vi "CODMn流程步骤.vi"() -> ()   [LabVIEW 2016]
panel:
  out "步骤时间/秒":T1={"步骤1时间"=2, "步骤2时间"=4, "步骤3时间"=2, "步骤4时间"=5, "步骤5时间"=6, "步骤6时间"=3, "步骤7时间"=4, "步骤8时间"=7, "步骤9时间"=8, "步骤10时间"=6}
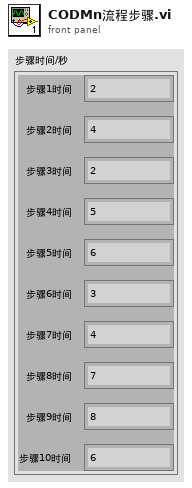
[diagram p1: front panel]
types:
  T1 = cluster{"步骤1时间":i32, "步骤2时间":i32, "步骤3时间":i32, "步骤4时间":i32, "步骤5时间":i32, "步骤6时间":i32, "步骤7时间":i32, "步骤8时间":i32, "步骤9时间":i32, "步骤10时间":i32}
  T2 = enum16{"步骤1", "步骤2", "步骤3", "步骤4", "步骤5", "步骤6", "步骤7", "步骤8", "步骤9", "步骤10"}
  T3 = cluster{"因子编码":u32, "单位":u16, "标样参考值":sgl, "水样数据时间":timestamp, "水样实测值":sgl, "水样数据标识":string, "标样数据时间":timestamp, "标样实测值":sgl, "标样数据标识":string, "空白数据时间":timestamp, "空白实测值":sgl, "空白数据标识":string, "零点核查数据时间":timestamp, "零点核查实测值":sgl, "零点核查数据标识":string, "跨度核查数据时间":timestamp, "跨度核查实测值":sgl, "跨度核查数据标识":string, "加标回收数据时间":timestamp, "加标回收实测值":sgl, "加标回收数据标识":string, "平行样数据时间":timestamp, "平行样实测值":sgl, "平行样数据标识":string}
  T4 = cluster{"系统时间":timestamp, "工作状态":u16, "测量模式":u16, "告警代码":enum16{"无告警", "缺试剂告警", "缺水样告警", "缺蒸馏水告警", "缺标液告警", "仪表漏液告警", "标定异常告警", "超量程告警", "加热异常", "低试剂预警", "超上限告警", "超下限告警", "仪表内部其他异常", "滴定异常告警", "电极异常告警", "量程切换告警", "参数设置告警", "PH电极电位异常", "电导率电极异常", "浊度光度异常", "溶解氧电极异常", "溶解氧光强异常", "温度异常告警", "PH异常告警", "溶解氧异常告警", "电导率异常告警", "浊度异常告警", "叶绿素异常告警", "藻密度异常告警", "蓝绿藻异常告警", "ORP异常告警", "氨氮异常告警", "清洁刷异常告警", "SD卡异常告警", "蓝牙异常告警", "Wifi异常告警", "流程异常告警"}, "故障代码":enum16{"无故障", "电机故障", "温度故障", "通讯故障", "滴定故障"}, "日志代码":u16, "软件版本":u16, "F0":sgl, "F1":sgl, "F2":sgl, "F3":sgl, "T":sgl, "H":sgl, "id":u16, "flowid":u16, "量程":u16}
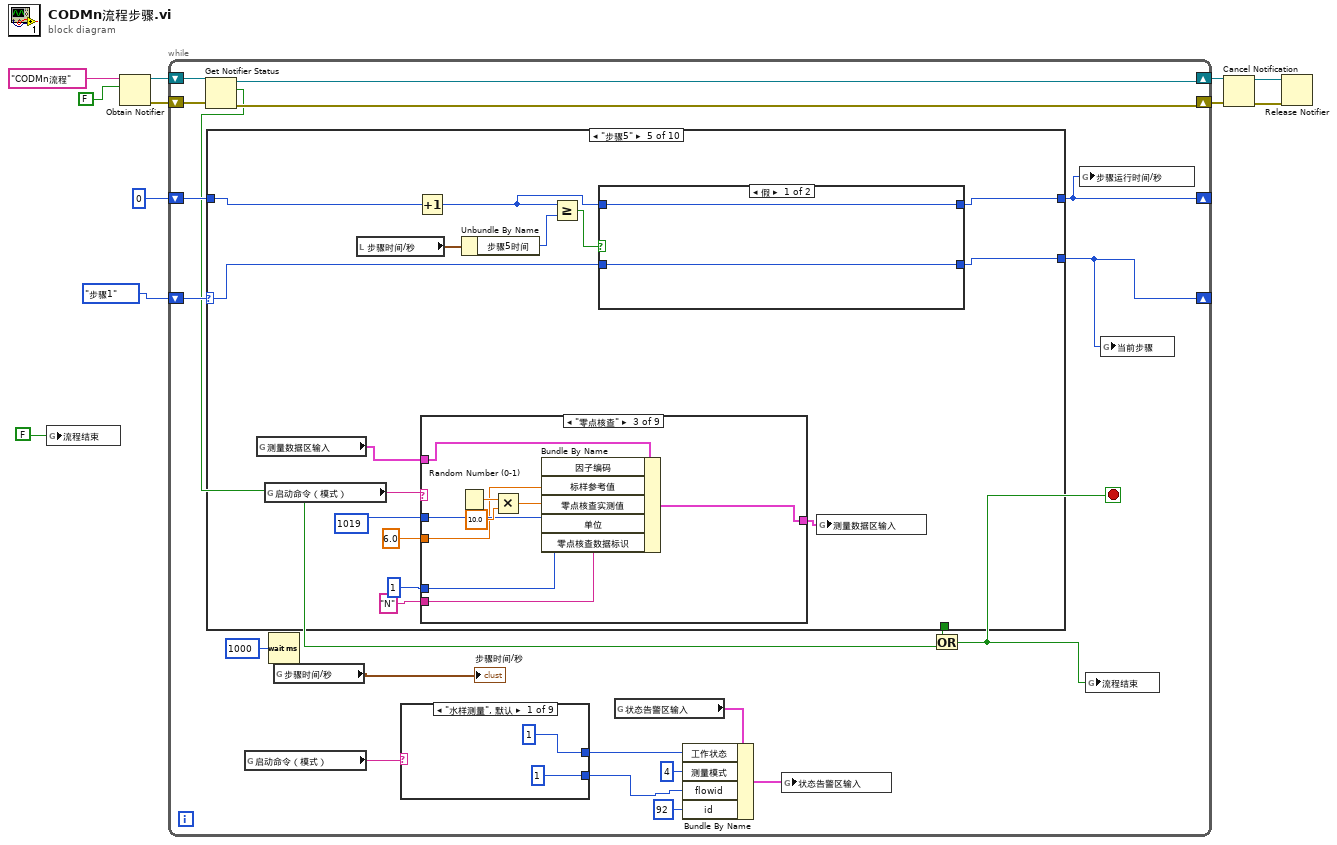
[diagram p0: block diagram]
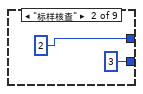
[diagram p2: hidden frame]
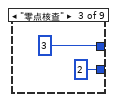
[diagram p3: hidden frame]
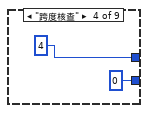
[diagram p4: hidden frame]
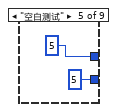
[diagram p5: hidden frame]
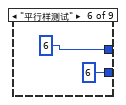
[diagram p6: hidden frame]
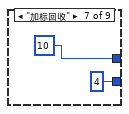
[diagram p7: hidden frame]
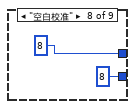
[diagram p8: hidden frame]
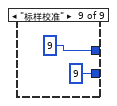
[diagram p9: hidden frame]
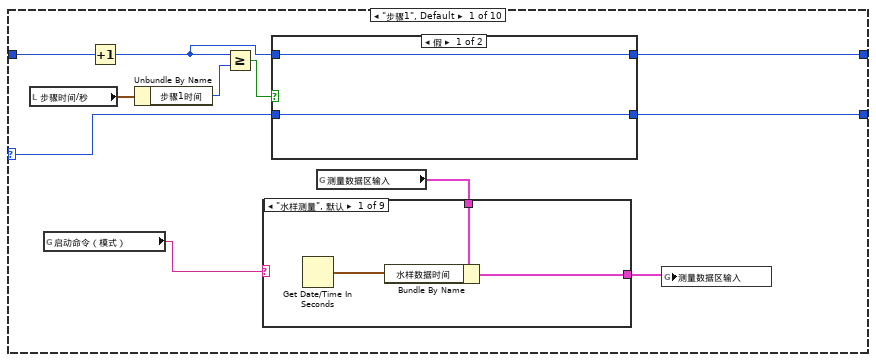
[diagram p10: hidden frame]
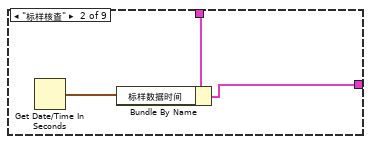
[diagram p11: hidden frame]
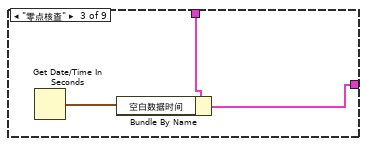
[diagram p12: hidden frame]
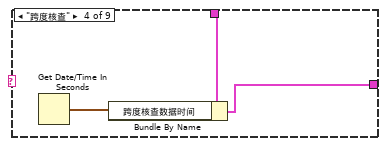
[diagram p13: hidden frame]
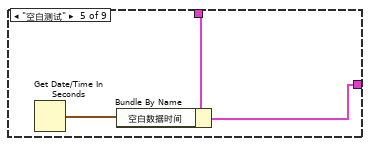
[diagram p14: hidden frame]
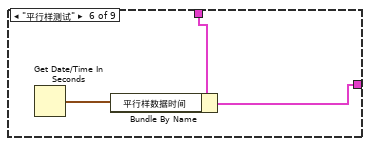
[diagram p15: hidden frame]
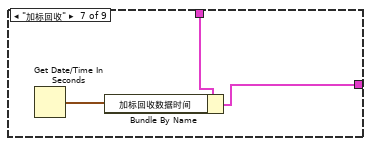
[diagram p16: hidden frame]
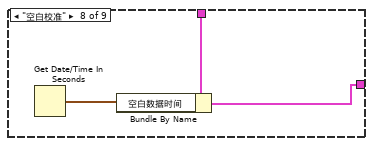
[diagram p17: hidden frame]
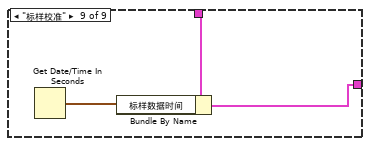
[diagram p18: hidden frame]
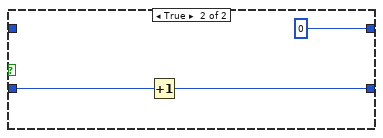
[diagram p19: hidden frame]
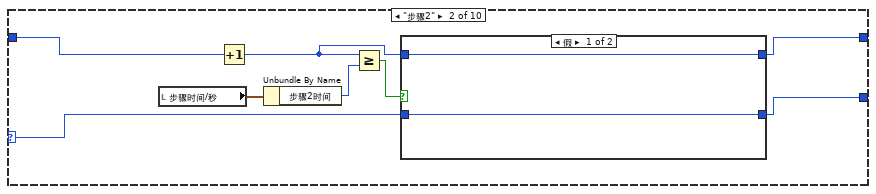
[diagram p20: hidden frame]
diagram:
  n1 = global write "CODMn全局.vi" "流程结束"(FALSE ("流程结束")) -> ()
  n2 = Obtain Notifier(name (unnamed)="CODMn流程" ("名称（未命名）"), notification data type=FALSE) -> (notifier out=w7:refnum<notifier>, error out=w6:errorcluster)  [unwired: 2 in, 1 out]
  n3 = while {
    shift-right: [w16] -> _
    shift-left: T2."步骤1" -> [w31]
    shift-right: [w17] -> _
    shift-left: 0 -> [w29]
    shift-right: [w25] -> w3
    shift-left: w7 -> [w27]
    shift-right: [w24] -> w2
    shift-left: w6 -> [w26]
    stop <- w18 stop-if-true
    n4 = Get Notifier Status(notifier=w27, error in (no error)=w26) -> (notifier out=w25:refnum<notifier>, current notification=w23:bool, error out=w24:errorcluster)  [unwired: 2 out]
    n5 = case shown="\"步骤5\"" w31 {
      selector: w31 -> [w54 w95 w108 w121 w141 w235 w248 w261 w274 w288]
      tunnel: [_ _ _ _ _ _ _ _ _ w285] -> w28
      tunnel: w29 -> [w60 w96 w109 w122 w142 w236 w249 w262 w275 w289]
      tunnel: [w56 w94 w107 w120 w140 w234 w247 w260 w273 w287] -> w17
      tunnel: [w53 w93 w106 w119 w139 w233 w246 w259 w272 w286] -> w16
      frame "步骤1", Default {
        n6 = local read "步骤时间/秒"() -> (w59:T1)
        n7 = global read "CODMn全局.vi" "启动命令（模式）"() -> (w50:string)
        n8 = Increment(x=w60) -> (x+1=w55:i32)
        n9 = Unbundle By Name(w59) -> ("步骤1时间"=w58:i32)
        n10 = Greater Or Equal?(x=w55, y=w58) -> (x >= y?=w57:bool)
        n11 = case shown="假" w57 {
          tunnel: [w89 0] -> w56
          tunnel: w55 -> [w89 _]
          tunnel: w54 -> [w88 w91]
          tunnel: [w88 w90] -> w53
          frame False {
          }
          frame True {
            n12 = Increment(x=w91) -> (x+1=w90:T2)
          }
        }
        n13 = global read "CODMn全局.vi" "测量数据区输入"() -> (w52:T3)
        n14 = case shown="\"水样测量\", 默认" w50 {
          tunnel: w52 -> [w62 w65 w68 w71 w74 w77 w80 w83 w86]
          tunnel: [w61 w64 w67 w70 w73 w76 w79 w82 w85] -> w51
          frame "水样测量", Default {
            n15 = Get Date/Time In Seconds() -> (seconds since 1Jan1904=w63:timestamp)
            n16 = Bundle By Name(cluster=w62, "水样数据时间"=w63) -> (w61:T3)
          }
          frame "标样核查" {
            n17 = Get Date/Time In Seconds() -> (seconds since 1Jan1904=w66:timestamp)
            n18 = Bundle By Name(cluster=w65, "标样数据时间"=w66) -> (w64:T3)
          }
          frame "零点核查" {
            n19 = Get Date/Time In Seconds() -> (seconds since 1Jan1904=w69:timestamp)
            n20 = Bundle By Name(cluster=w68, "空白数据时间"=w69) -> (w67:T3)
          }
          frame "跨度核查" {
            n21 = Get Date/Time In Seconds() -> (seconds since 1Jan1904=w72:timestamp)
            n22 = Bundle By Name(cluster=w71, "跨度核查数据时间"=w72) -> (w70:T3)
          }
          frame "空白测试" {
            n23 = Get Date/Time In Seconds() -> (seconds since 1Jan1904=w75:timestamp)
            n24 = Bundle By Name(cluster=w74, "空白数据时间"=w75) -> (w73:T3)
          }
          frame "平行样测试" {
            n25 = Get Date/Time In Seconds() -> (seconds since 1Jan1904=w78:timestamp)
            n26 = Bundle By Name(cluster=w77, "平行样数据时间"=w78) -> (w76:T3)
          }
          frame "加标回收" {
            n27 = Get Date/Time In Seconds() -> (seconds since 1Jan1904=w81:timestamp)
            n28 = Bundle By Name(cluster=w80, "加标回收数据时间"=w81) -> (w79:T3)
          }
          frame "空白校准" {
            n29 = Get Date/Time In Seconds() -> (seconds since 1Jan1904=w84:timestamp)
            n30 = Bundle By Name(cluster=w83, "空白数据时间"=w84) -> (w82:T3)
          }
          frame "标样校准" {
            n31 = Get Date/Time In Seconds() -> (seconds since 1Jan1904=w87:timestamp)
            n32 = Bundle By Name(cluster=w86, "标样数据时间"=w87) -> (w85:T3)
          }
        }
        n33 = global write "CODMn全局.vi" "测量数据区输入"(w51) -> ()
      }
      frame "步骤2" {
        n34 = local read "步骤时间/秒"() -> (w100:T1)
        n35 = Increment(x=w96) -> (x+1=w97:i32)
        n36 = Unbundle By Name(w100) -> ("步骤2时间"=w99:i32)
        n37 = Greater Or Equal?(x=w97, y=w99) -> (x >= y?=w98:bool)
        n38 = case shown="假" w98 {
          tunnel: [w102 0] -> w94
          tunnel: w97 -> [w102 _]
          tunnel: w95 -> [w101 w104]
          tunnel: [w101 w103] -> w93
          frame False {
          }
          frame True {
            n39 = Increment(x=w104) -> (x+1=w103:T2)
          }
        }
      }
      frame "步骤3" {
        n40 = local read "步骤时间/秒"() -> (w113:T1)
        n41 = Increment(x=w109) -> (x+1=w110:i32)
        n42 = Unbundle By Name(w113) -> ("步骤3时间"=w112:i32)
        n43 = Greater Or Equal?(x=w110, y=w112) -> (x >= y?=w111:bool)
        n44 = case shown="假" w111 {
          tunnel: [w115 0] -> w107
          tunnel: w110 -> [w115 _]
          tunnel: w108 -> [w114 w117]
          tunnel: [w114 w116] -> w106
          frame False {
          }
          frame True {
            n45 = Increment(x=w117) -> (x+1=w116:T2)
          }
        }
      }
      frame "步骤4" {
        n46 = local read "步骤时间/秒"() -> (w126:T1)
        n47 = Increment(x=w122) -> (x+1=w123:i32)
        n48 = Unbundle By Name(w126) -> ("步骤4时间"=w125:i32)
        n49 = Greater Or Equal?(x=w123, y=w125) -> (x >= y?=w124:bool)
        n50 = case shown="假" w124 {
          tunnel: [w128 0] -> w120
          tunnel: w123 -> [w128 _]
          tunnel: w121 -> [w127 w130]
          tunnel: [w127 w129] -> w119
          frame False {
          }
          frame True {
            n51 = Increment(x=w130) -> (x+1=w129:T2)
          }
        }
      }
      frame "步骤5" {
        n52 = global read "CODMn全局.vi" "测量数据区输入"() -> (w133:T3)
        n53 = global read "CODMn全局.vi" "启动命令（模式）"() -> (w134:string)
        n54 = local read "步骤时间/秒"() -> (w146:T1)
        n55 = Increment(x=w142) -> (x+1=w143:i32)
        n56 = case shown="\"零点核查\"" w134 {
          tunnel: u32 1019 ("因子编码") -> [w151 w161 w170 w179 w188 w197 w206 w215 w224]
          tunnel: sgl 6.0 ("标样参考值") -> [w150 w160 w169 w177 w186 w195 w204 w213 w222]
          tunnel: u16 1 ("单位") -> [w149 w159 w168 w178 w187 w196 w205 w214 w223]
          tunnel: "N" -> [w152 w158 w167 w176 w185 w194 w203 w212 w221]
          tunnel: w133 -> [w148 w157 w166 w175 w184 w192 w202 w211 w220]
          tunnel: [w147 w156 w165 w174 w183 w193 w201 w210 w219] -> w132
          frame "水样测量", Default {
            n57 = Random Number (0-1)() -> (number: 0 to 1=w153:dbl)
            n58 = Multiply(x=w153, y=10.0 ("数字(0-1)")) -> (x*y=w155:dbl)
            n59 = Bundle By Name(cluster=w148, "因子编码"=w151, "标样参考值"=w150, "水样实测值"=w155, "单位"=w149, "水样数据标识"=w152) -> (w147:T3)
          }
          frame "标样核查" {
            n60 = Random Number (0-1)() -> (number: 0 to 1=w162:dbl)
            n61 = Multiply(x=w162, y=10.0 ("数字(0-1)")) -> (x*y=w164:dbl)
            n62 = Bundle By Name(cluster=w157, "因子编码"=w161, "标样参考值"=w160, "标样实测值"=w164, "单位"=w159, "标样数据标识"=w158) -> (w156:T3)
          }
          frame "零点核查" {
            n63 = Random Number (0-1)() -> (number: 0 to 1=w171:dbl)
            n64 = Multiply(x=w171, y=10.0 ("数字(0-1)")) -> (x*y=w173:dbl)
            n65 = Bundle By Name(cluster=w166, "因子编码"=w170, "标样参考值"=w169, "零点核查实测值"=w173, "单位"=w168, "零点核查数据标识"=w167) -> (w165:T3)
          }
          frame "跨度核查" {
            n66 = Random Number (0-1)() -> (number: 0 to 1=w180:dbl)
            n67 = Multiply(x=w180, y=10.0 ("数字(0-1)")) -> (x*y=w182:dbl)
            n68 = Bundle By Name(cluster=w175, "因子编码"=w179, "标样参考值"=w177, "跨度核查实测值"=w182, "单位"=w178, "跨度核查数据标识"=w176) -> (w174:T3)
          }
          frame "空白测试" {
            n69 = Random Number (0-1)() -> (number: 0 to 1=w189:dbl)
            n70 = Multiply(x=w189, y=10.0 ("数字(0-1)")) -> (x*y=w191:dbl)
            n71 = Bundle By Name(cluster=w184, "因子编码"=w188, "标样参考值"=w186, "空白实测值"=w191, "单位"=w187, "空白数据标识"=w185) -> (w183:T3)
          }
          frame "平行样测试" {
            n72 = Random Number (0-1)() -> (number: 0 to 1=w198:dbl)
            n73 = Multiply(x=w198, y=10.0 ("数字(0-1)")) -> (x*y=w200:dbl)
            n74 = Bundle By Name(cluster=w192, "因子编码"=w197, "标样参考值"=w195, "平行样实测值"=w200, "单位"=w196, "平行样数据标识"=w194) -> (w193:T3)
          }
          frame "加标回收" {
            n75 = Random Number (0-1)() -> (number: 0 to 1=w207:dbl)
            n76 = Multiply(x=w207, y=10.0 ("数字(0-1)")) -> (x*y=w209:dbl)
            n77 = Bundle By Name(cluster=w202, "因子编码"=w206, "标样参考值"=w204, "加标回收实测值"=w209, "单位"=w205, "加标回收数据标识"=w203) -> (w201:T3)
          }
          frame "空白校准" {
            n78 = Random Number (0-1)() -> (number: 0 to 1=w216:dbl)
            n79 = Multiply(x=w216, y=10.0 ("数字(0-1)")) -> (x*y=w218:dbl)
            n80 = Bundle By Name(cluster=w211, "因子编码"=w215, "标样参考值"=w213, "空白实测值"=w218, "单位"=w214, "跨度核查数据标识"=w212) -> (w210:T3)
          }
          frame "标样校准" {
            n81 = Random Number (0-1)() -> (number: 0 to 1=w225:dbl)
            n82 = Multiply(x=w225, y=10.0 ("数字(0-1)")) -> (x*y=w227:dbl)
            n83 = Bundle By Name(cluster=w220, "因子编码"=w224, "标样参考值"=w222, "标样实测值"=w227, "单位"=w223, "跨度核查数据标识"=w221) -> (w219:T3)
          }
        }
        n84 = Unbundle By Name(w146) -> ("步骤5时间"=w145:i32)
        n85 = Greater Or Equal?(x=w143, y=w145) -> (x >= y?=w144:bool)
        n86 = case shown="假" w144 {
          tunnel: [w229 0] -> w140
          tunnel: w143 -> [w229 _]
          tunnel: w141 -> [w228 w231]
          tunnel: [w228 w230] -> w139
          frame False {
          }
          frame True {
            n87 = Increment(x=w231) -> (x+1=w230:T2)
          }
        }
        n88 = global write "CODMn全局.vi" "测量数据区输入"(w132) -> ()
      }
      frame "步骤6" {
        n89 = local read "步骤时间/秒"() -> (w240:T1)
        n90 = Increment(x=w236) -> (x+1=w237:i32)
        n91 = Unbundle By Name(w240) -> ("步骤6时间"=w239:i32)
        n92 = Greater Or Equal?(x=w237, y=w239) -> (x >= y?=w238:bool)
        n93 = case shown="假" w238 {
          tunnel: [w242 0] -> w234
          tunnel: w237 -> [w242 _]
          tunnel: w235 -> [w241 w244]
          tunnel: [w241 w243] -> w233
          frame False {
          }
          frame True {
            n94 = Increment(x=w244) -> (x+1=w243:T2)
          }
        }
      }
      frame "步骤7" {
        n95 = local read "步骤时间/秒"() -> (w253:T1)
        n96 = Increment(x=w249) -> (x+1=w250:i32)
        n97 = Unbundle By Name(w253) -> ("步骤7时间"=w252:i32)
        n98 = Greater Or Equal?(x=w250, y=w252) -> (x >= y?=w251:bool)
        n99 = case shown="假" w251 {
          tunnel: [w255 0] -> w247
          tunnel: w250 -> [w255 _]
          tunnel: w248 -> [w254 w257]
          tunnel: [w254 w256] -> w246
          frame False {
          }
          frame True {
            n100 = Increment(x=w257) -> (x+1=w256:T2)
          }
        }
      }
      frame "步骤8" {
        n101 = local read "步骤时间/秒"() -> (w266:T1)
        n102 = Increment(x=w262) -> (x+1=w263:i32)
        n103 = Unbundle By Name(w266) -> ("步骤8时间"=w265:i32)
        n104 = Greater Or Equal?(x=w263, y=w265) -> (x >= y?=w264:bool)
        n105 = case shown="假" w264 {
          tunnel: [w268 0] -> w260
          tunnel: w263 -> [w268 _]
          tunnel: w261 -> [w267 w270]
          tunnel: [w267 w269] -> w259
          frame False {
          }
          frame True {
            n106 = Increment(x=w270) -> (x+1=w269:T2)
          }
        }
      }
      frame "步骤9" {
        n107 = local read "步骤时间/秒"() -> (w279:T1)
        n108 = Increment(x=w275) -> (x+1=w276:i32)
        n109 = Unbundle By Name(w279) -> ("步骤9时间"=w278:i32)
        n110 = Greater Or Equal?(x=w276, y=w278) -> (x >= y?=w277:bool)
        n111 = case shown="假" w277 {
          tunnel: [w281 0] -> w273
          tunnel: w276 -> [w281 _]
          tunnel: w274 -> [w280 w283]
          tunnel: [w280 w282] -> w272
          frame False {
          }
          frame True {
            n112 = Increment(x=w283) -> (x+1=w282:T2)
          }
        }
      }
      frame "步骤10" {
        n113 = local read "步骤时间/秒"() -> (w293:T1)
        n114 = Increment(x=w289) -> (x+1=w290:i32)
        n115 = Unbundle By Name(w293) -> ("步骤10时间"=w292:i32)
        n116 = Greater Or Equal?(x=w290, y=w292) -> (x >= y?=w291:bool)
        n117 = case shown="真" w291 {
          tunnel: [w295 0] -> w287
          tunnel: w290 -> [w295 _]
          tunnel: w288 -> [w294 w298]
          tunnel: [w294 w297] -> w286
          tunnel: [_ TRUE] -> w285
          frame False {
          }
          frame True {
            n118 = Increment(x=w298) -> (x+1=w297:T2)
          }
        }
      }
    }
    n119 = global read "CODMn全局.vi" "启动命令（模式）"() -> (w15:string)
    n120 = Wait (ms)(milliseconds to wait=u32 1000 ("等待时间（毫秒）")) -> ()  [unwired: 1 out]
    n121 = global read "CODMn全局.vi" "步骤时间/秒"() -> (→"步骤时间/秒":T1)
    n122 = case shown="\"水样测量\", 默认" w15 {
      tunnel: [u16 1 ("工作状态") u16 2 ("工作状态") u16 3 ("工作状态") u16 4 ("工作状态") u16 5 ("工作状态") u16 6 ("工作状态") u16 10 ("工作状态") u16 8 ("工作状态") u16 9 ("工作状态")] -> w21
      tunnel: [u16 1 ("工作状态") u16 3 ("工作状态") u16 2 ("工作状态") u16 0 ("工作状态") u16 5 ("工作状态") u16 6 ("工作状态") u16 4 ("工作状态") u16 8 ("工作状态") u16 9 ("工作状态")] -> w19
      frame "水样测量", Default {
      }
      frame "标样核查" {
      }
      frame "零点核查" {
      }
      frame "跨度核查" {
      }
      frame "空白测试" {
      }
      frame "平行样测试" {
      }
      frame "加标回收" {
      }
      frame "空白校准" {
      }
      frame "标样校准" {
      }
    }
    n123 = global read "CODMn全局.vi" "状态告警区输入"() -> (w13:T4)
    n124 = Bundle By Name(cluster=w13, "工作状态"=w21, "测量模式"=u16 4, "flowid"=w19, "id"=u16 92) -> (w12:T4)
    n125 = global write "CODMn全局.vi" "状态告警区输入"(w12) -> ()
    n126 = Or(x=w28, y=w23) -> (x .or. y?=w18:bool)
    n127 = global write "CODMn全局.vi" "步骤运行时间/秒"(w17) -> ()
    n128 = global write "CODMn全局.vi" "流程结束"(w18) -> ()
    n129 = global write "CODMn全局.vi" "当前步骤"(w16) -> ()
  }
  n130 = Cancel Notification(0:w3, 3:w2) -> (8:w5:refnum<notifier>, 11:w4:errorcluster)  [unwired: 1 out]
  n131 = Release Notifier(notifier=w5, error in (no error)=w4) -> ()  [unwired: 1 in, 3 out]
